vi "Preview.vi"(8 "error in (no error)":errorcluster, 10 "collect dependencies? (F)":bool, 11 "EXE in":refnum<class "NI_AB_API_EXE.lvclass">) -> (0 "error out":errorcluster, 1 "Dependencies":T1[](array[typedef]), 2 "GeneratedFiles":path[](array[path]), 3 "EXE out":refnum<class "NI_AB_API_EXE.lvclass">)   [LabVIEW 2020, in "NI_AB_API_EXE.lvclass"]
uses:
  <vilib>/AppBuilder/AB_API/EXE/NI_AB_API_EXE.lvclass
  <vilib>/AppBuilder/AB_Dependency.ctl
  <vilib>/Utility/lvfile.llb/LVFileType.ctl
  <vilib>/AppBuilder/AB_API/Application/NI_AB_API_Application.lvclass
  <vilib>/Utility/lvfile.llb/NI_FileType.lvlib
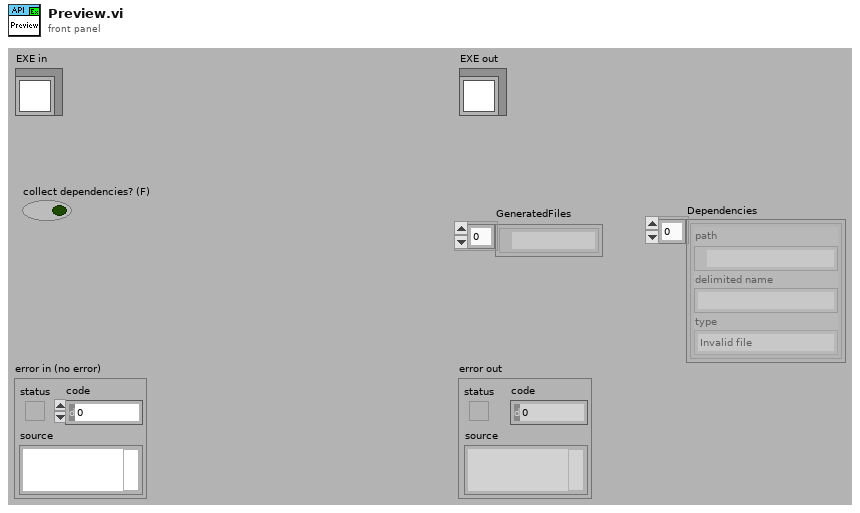
[diagram p1: front panel]
types:
  T1 = typedef "AB_Dependency.ctl" = cluster{"path":path, "delimited name":string, "type":T2}
  T2 = typedef "NI_FileType.lvlib/LVFileType.ctl" = enum32{"Invalid file", "Unknown type", "Instrument", "Control", "Polymorphic VI", "Project", "Library", "LVClass", "XControl", "XNode", "Shared library", ".NET assembly", "ActiveX interface", "CIN", "Run-time menu", "Palette menu", "Help file", "LLB", "XNode Edit Dependency", "Class Private Data Control", "Statechart", "MathScript .m file", "Ladder Diagram", "LVLibp", "XNode Build Dependency"}
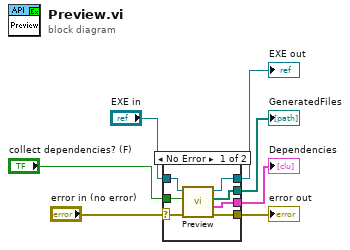
[diagram p0: block diagram]
diagram:
  n1 = case shown="No Error" "error in (no error)" {
    selector: "error in (no error)" -> [w13 w16]
    tunnel: [w11 w16] -> w6
    tunnel: [w12 w15] -> w4
    tunnel: "EXE in" -> [w14 w15]
    tunnel: [w10 _] -> w3
    tunnel: [w9 _] -> w2
    tunnel: "collect dependencies? (F)" -> [w8 _]
    frame No Error {
      n2 = call-parent "Preview.vi"("error in (no error)"=w13, "collect dependencies? (F)"=w8, "Build in"=w14) -> ("error out"=w11:errorcluster, "Dependencies"=w9:T1[], "GeneratedFiles"=w10:path[], "Build out"=w12:refnum<class "NI_AB_API_EXE.lvclass">)  [unwired: 5 in]
    }
    frame Error {
    }
  }
  "error out" <- w6
  "EXE out" <- w4
  "GeneratedFiles" <- w3
  "Dependencies" <- w2
